vi "pr2b.vi"() -> ()   [LabVIEW 2013]
uses:
  <vilib>/Platform/TimedLoop/XDataNode/timing_clust.ctl
  <vilib>/Platform/TimedLoop/XDataNode/nitl_modes.ctl
  <vilib>/Platform/TimedLoop/XDataNode/wakeup.ctl
  <vilib>/DAQmx/write.llb/DAQmx Write (Counter Frequency 1Chan 1Samp).vi
  <vilib>/DAQmx/read.llb/DAQmx Read (Counter DBL 1Chan 1Samp).vi
  <vilib>/DAQmx/write.llb/DAQmx Write (Digital Bool 1Line 1Point).vi
  <vilib>/DAQmx/create/channels.llb/DAQmx Create Channel (CI-Position-Angular Encoder).vi
  <vilib>/DAQmx/create/channels.llb/DAQmx Create Channel (DO-Digital Output).vi
  <vilib>/DAQmx/create/channels.llb/DAQmx Create Channel (CO-Pulse Generation-Frequency).vi
  <vilib>/DAQmx/configure/timing.llb/DAQmx Timing (Implicit).vi
  <vilib>/DAQmx/miscellaneous.llb/DAQmx Fill In Error Info.vi
  <vilib>/platform/TimedLoop/XDataNode/XDataNode.xnode
  <vilib>/Platform/TimedLoop/XDataNode/XDNodeRunTimeDep.lvlib
panel:
  out "Error":errorcluster
  out "Y max":dbl format="%0.2f"
  out "RPM":waveform(dbl)(graph)
  in  "Numero de ciclos de \nPWM por periodo de muestreo (N)":dbl=5.0
  in  "counter":tag="Dev1/ctr0"
  out "Señales Normalizadas":waveform(dbl)[](graph)
  out "Señal de entrada (DC)":waveform(dbl)(graph)
  in  "Duración de los ceros":dbl=1.0
  in  "Duracion de ciclo":dbl=30.0
  in  "Periodo de muestreo (seg)":dbl=0.01
  in  "lines":tag="Dev1/port0/line0"
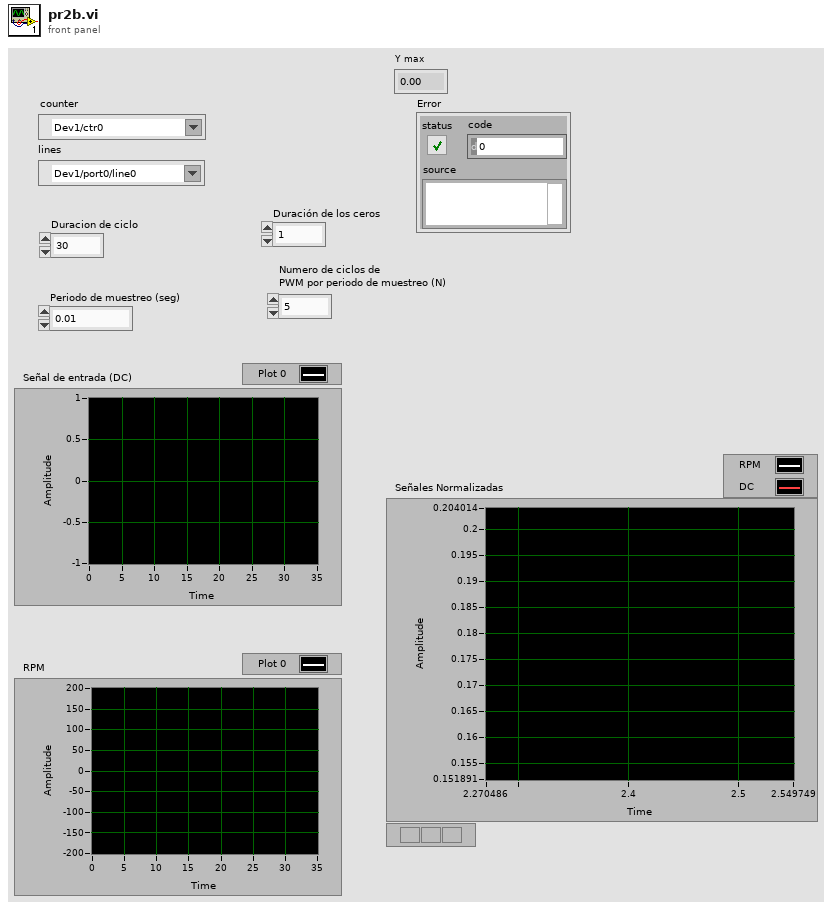
[diagram p1: front panel]
types:
  T1 = typedef "XDNodeRunTimeDep.lvlib/timing_clust.ctl" = cluster{"Expected End [f-1]":u64, "Actual End [f-1]":u64, "Finished Late? [f-1]":bool, "Expected End [i-1]":u64, "Actual End [i-1]":u64, "Finished Late? [i-1]":bool, "Expected Start [i]":u64, "Actual Start [i]":u64, "Expected Start [f]":u64, "Actual Start [f]":u64, "Source Name":string, "Structure Name":string, "Period":i64, "Deadline":i64, "Offset":i64, "Start":i64, "Priority":i32, "Timeout":i32, "Mode":T2, "Wakeup Reason":T3, "Error":errorcluster, "Source Type":string, "Secondary Source Type":string, "Global End Time":u64, "Global Start Time":u64, "Frame Duration":u64, "Iteration Duration":u64, "Assigned CPU":i32, "I/O Scan Engine Mode":u32}
  T2 = typedef "XDNodeRunTimeDep.lvlib/nitl_modes.ctl" = enum32{"No Change", "Process missed periods, maintain original phase", "Discard missed periods, maintain original phase", "Process missed periods, ignore original phase", "Discard missed periods, ignore original phase"}
  T3 = typedef "XDNodeRunTimeDep.lvlib/wakeup.ctl" = enum32{"Normal", "Aborted", "Asynchronous wakeup", "Timing source error", "Timed loop error", "Timeout"}
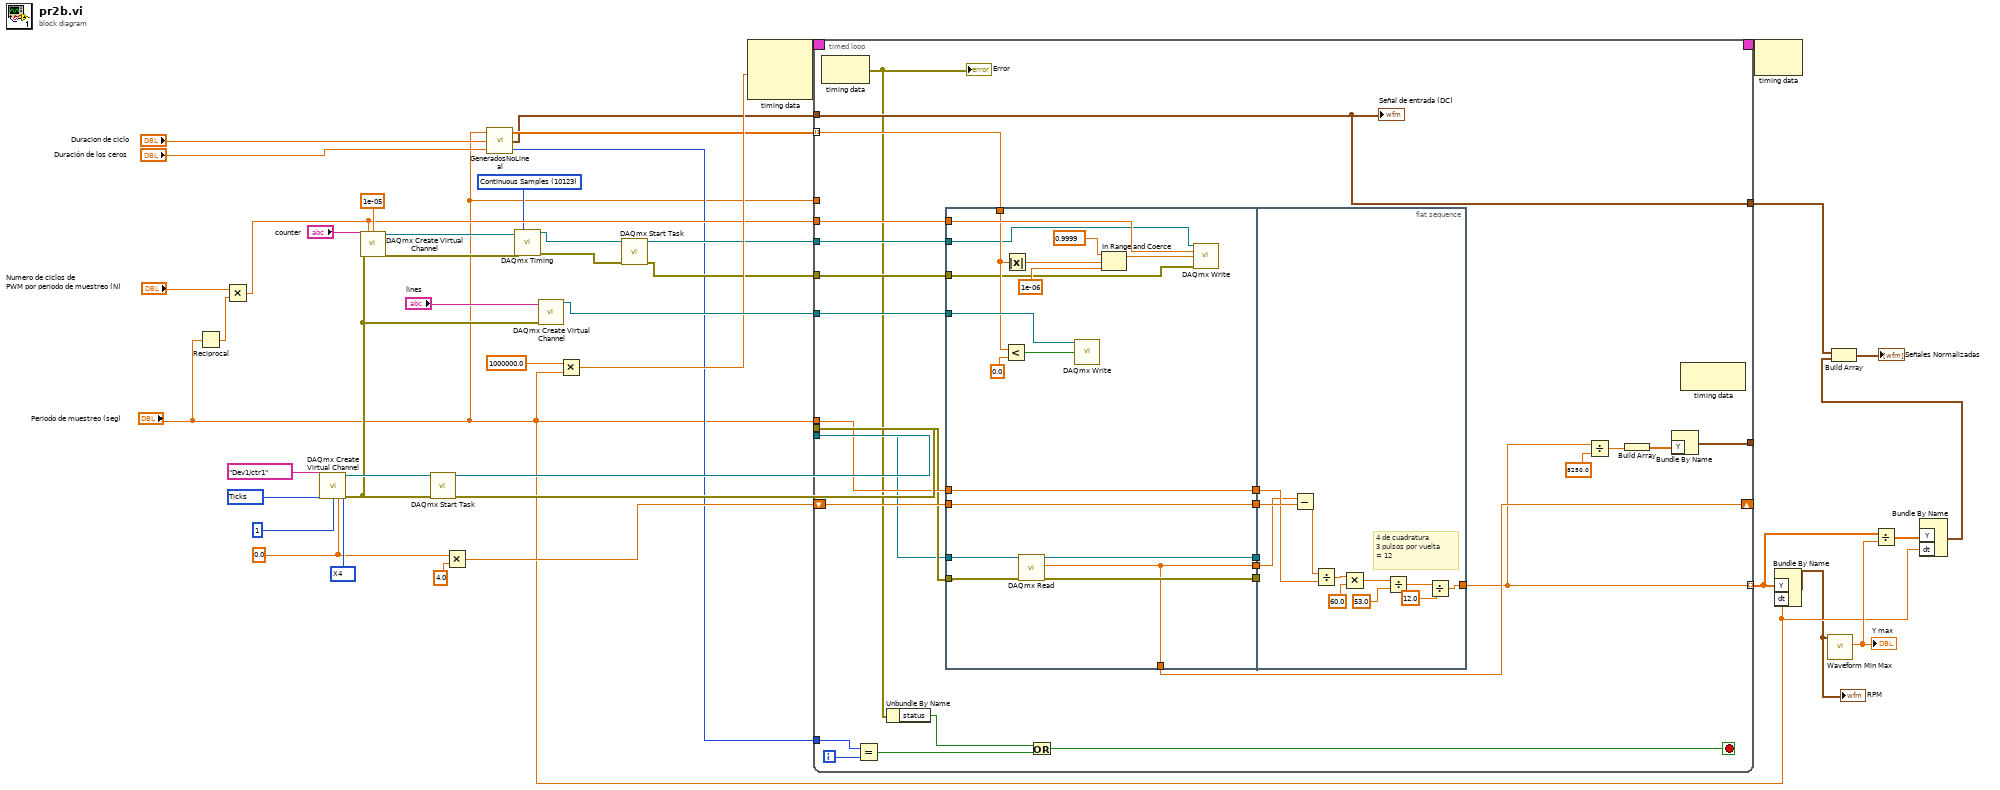
[diagram p0: block diagram]
diagram:
  w10 = 10123 items=["Finite Samples"=10178, "Continuous Samples"=10123, "Hardware Timed Single Point"=12522] ("sample mode")
  w37 = 10092 items=["X1"=10090, "X2"=10091, "X4"=10092, "Two Pulse Counting"=10313] ("decoding type")
  w32 = 0.0 ("initial angle")
  w39 = 10304 items=["Degrees"=10146, "Radians"=10273, "Ticks"=10304, "From Custom Scale"=10065] ("units")
  n1 = Reciprocal(x="Periodo de muestreo (seg)") -> (1/x=w17:dbl)
  n2 = Multiply(x="Numero de ciclos de \nPWM por periodo de muestreo (N)", y=w17) -> (x*y=w18:dbl)
  n3 = call-poly <vilib>:"DAQmx Create Virtual Channel.vi"("counter"=tag "Dev1/ctr1", "decoding type"=w37, "units"=w39, "pulses per revolution"=u32 1, "initial angle"=w32) -> ("task out"=w36:refnum<k21>, "error out"=w21:errorcluster)  [unwired: 9 in]
  n4 = call-poly <vilib>:"DAQmx Create Virtual Channel.vi"("frequency"=w18, "duty cycle"=1e-05, "counter"="counter", "error in"=w21) -> ("task out"=w16:refnum<k21>, "error out"=w13:errorcluster)  [unwired: 10 in]
  n5 = call <vilib>:"DAQmx Start Task.vi"("task/channels in"=w36, "error in"=w21) -> ("task out"=w35:refnum<k21>, "error out"=w34:errorcluster)  [unwired: 12 in]
  n6 = Multiply(x=w32, y=4.0) -> (x*y=w19:dbl)
  n7 = call "GeneradosNoLineal.vi"("Duración de los ceros"="Duración de los ceros", "Duración de ciclo (s)"="Duracion de ciclo", "Periodo de muestreo"="Periodo de muestreo (seg)") -> ("Numero de muestras"=w7:i32, "Waveform Graph 2"=w20:waveform(dbl), "Señal No linealidad"=w25:dbl[])
  n8 = call-poly <vilib>:"DAQmx Timing.vi"("task/channels in"=w16, "sample mode"=w10, "error in"=w13) -> ("task out"=w15:refnum<k21>, "error out"=w12:errorcluster)  [unwired: 11 in]
  n9 = call-poly <vilib>:"DAQmx Create Virtual Channel.vi"("lines"="lines", "error in"=w21) -> ("task out"=w27:refnum<k21>)  [unwired: 12 in, 1 out]
  n10 = Multiply(x=1000000.0, y="Periodo de muestreo (seg)") -> (x*y=w26:dbl)
  n11 = call <vilib>:"DAQmx Start Task.vi"("task/channels in"=w15, "error in"=w12) -> ("task out"=w14:refnum<k21>, "error out"=w11:errorcluster)  [unwired: 12 in]
  n12 = node-c288(w26) -> (w41:T1)  [unwired: 2 in]
  n13 = timed-loop {
    timing: w41 -> [_]
    timing-out: [_] -> w40
    shift-right: [w60] -> _
    shift-left: w19 -> [w69]
    tunnel: w35 -> [w62]
    tunnel: w34 -> [w63]
    tunnel: "Periodo de muestreo (seg)" -> [w68]
    tunnel: w25 -> [w56] mode=indexing
    tunnel: "Periodo de muestreo (seg)" -> [_]
    tunnel: w27 -> [w65]
    tunnel: w20 -> [w53]
    tunnel: w18 -> [w57]
    tunnel: w14 -> [w55]
    tunnel: w11 -> [w54]
    tunnel: [w51] -> w6 mode=indexing
    tunnel: [w53] -> w9
    tunnel: w7 -> [w52]
    tunnel: [w47] -> _
    i -> [w58]
    stop <- w43 stop-if-true
    n14 = node-c288() -> (w46:errorcluster)  [unwired: 1 in]
    "Error" <- w46
    n15 = Equal?(x=w52, y=w58) -> (x = y?=w45:bool)
    n16 = Unbundle By Name(w46) -> ("status"=w44:bool)
    n17 = flat-sequence {
      tunnel: w68 -> [w86]
      tunnel: w69 -> [w87]
      tunnel: [w87] -> w67
      tunnel: [w86] -> w66
      tunnel: w65 -> [w81]
      tunnel: [w78] -> w64
      tunnel: w63 -> [w77]
      tunnel: w62 -> [w76]
      tunnel: [w75] -> w61
      tunnel: [w74] -> w60
      tunnel: [w74] -> w59
      tunnel: w57 -> [w73]
      tunnel: w56 -> [w72]
      tunnel: w55 -> [w71]
      tunnel: w54 -> [w70]
      tunnel: [w89] -> w51
      tunnel: w67 -> [w98]
      tunnel: w66 -> [w92]
      tunnel: w64 -> [_]
      tunnel: w61 -> [_]
      tunnel: w59 -> [w91]
      frame #0 {
        n18 = Less?(x=w72, y=0.0) -> (x < y?=w79:bool)
        n19 = Absolute Value(x=w72) -> (abs(x)=w83:dbl)
        n20 = call-poly <vilib>:"DAQmx Read.vi"("task/channels in"=w76, "error in"=w77) -> ("task out"=w75:refnum<k21>, "data"=w74:dbl, "error out"=w78:errorcluster)  [unwired: 11 in]
        n21 = call-poly <vilib>:"DAQmx Write.vi"("task/channels in"=w81, "data"=w79) -> ()  [unwired: 11 in, 3 out]
        n22 = In Range and Coerce(upper limit=0.9999, x=w83, lower limit=1e-06) -> (coerced(x)=w82:dbl)  [unwired: 1 out]
        n23 = call-poly <vilib>:"DAQmx Write.vi"("task/channels in"=w71, "frequency"=w73, "duty cycle"=w82, "error in"=w70) -> ()  [unwired: 9 in, 3 out]
      }
      frame #1 {
        # "4 de cuadratura\n3 pulsos por vuelta\n= 12"
        n24 = Subtract(x=w91, y=w98) -> (x-y=w97:dbl)
        n25 = Divide(x=w97, y=w92) -> (x/y=w96:dbl)
        n26 = Multiply(x=w96, y=60.0) -> (x*y=w94:dbl)
        n27 = Divide(x=w94, y=53.0) -> (x/y=w90:dbl)
        n28 = Divide(x=w90, y=12.0) -> (x/y=w89:dbl)
      }
    }
    n29 = Or(x=w44, y=w45) -> (x .or. y?=w43:bool)
    n30 = Divide(x=w51, y=8250.0) -> (x/y=w49:dbl)
    n31 = Build Array(w49) -> (w48:dbl[])
    n32 = Bundle By Name("Y"=w48) -> (w47:waveform(dbl))  [unwired: 1 in]
    n33 = node-c288() -> ()  [unwired: 1 in, 1 out]
    "Señal de entrada (DC)" <- w53
  }
  n34 = node-c288(w40) -> ()  [unwired: 1 out]
  n35 = Bundle By Name("Y"=w6, "dt"="Periodo de muestreo (seg)") -> (w1:waveform(dbl))  [unwired: 1 in]
  "RPM" <- w1
  n36 = call <vilib>:"Waveform Min Max.vi"("waveform in"=w1) -> ("Y max"=w5:dbl)  [unwired: 5 in, 5 out]
  "Y max" <- w5
  n37 = Divide(x=w6, y=w5) -> (x/y=w4:dbl[])
  n38 = Bundle By Name("Y"=w4, "dt"="Periodo de muestreo (seg)") -> (w2:waveform(dbl))  [unwired: 1 in]
  n39 = Build Array(w9, w2) -> (→"Señales Normalizadas":waveform(dbl)[])
